vi "WaveFile_Create.vi"(0 "reference in":refnum<class "WaveFile.lvclass">, 5 "error in (no error)":errorcluster, 6 "Time Data":refnum<class "GSwFormDSP.lvclass">, 7 "Application Name":string, 9 "State Queue":string[](array[string])) -> (14 "reference out":refnum<class "WaveFile.lvclass">, 19 "error out":errorcluster)   [LabVIEW 2020, in "WaveFile.lvclass"]
doc: "Constructor."
uses:
  WaveFile.lvclass
  C:/Program Files/National Instruments/LabVIEW 2020/vi.lib/addons/_AddQ/G#Object/G#Object.lvclass
  C:/Users/fcharett/docsWork/coding/20SPWB/C/Users/fcharett/docsWork/coding/LabVIEW/API/Generic Utilities_class/Generic Utilities.lvclass
  API/GSwFormDSP_class/GSwFormDSP.lvclass
  <vilib>/addons/_AddQ/G#Object/G#Object.lvclass
  API/Generic Utilities_class/Generic Utilities.lvclass
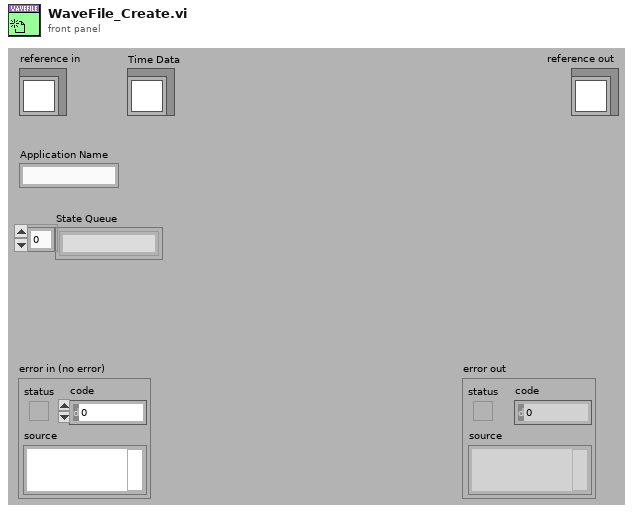
[diagram p1: front panel]
types:
  T1 = typedef "WaveFile.lvclass/ObjectAttributesRef.ctl" = refnum<data-value>
  T2 = typedef "WaveFile.lvclass/ObjectAttributes.ctl" = cluster{"Time Data":refnum<class "GSwFormDSP.lvclass">, "New Time Data Obj?":bool, "NIST File Header":T3}
  T3 = typedef "WaveFile.lvclass/NIST File Header.ctl" = cluster{"Version":string, "Header Nb Bytes":i32, "Nb Samples":i32, "Nb Bytes/sample":i32, "Nb Channels":i32, "byte order":enum16{"big-endian, network order", "native, host order", "little-endian"}, "Fs":dbl, "Valid Header?":bool}
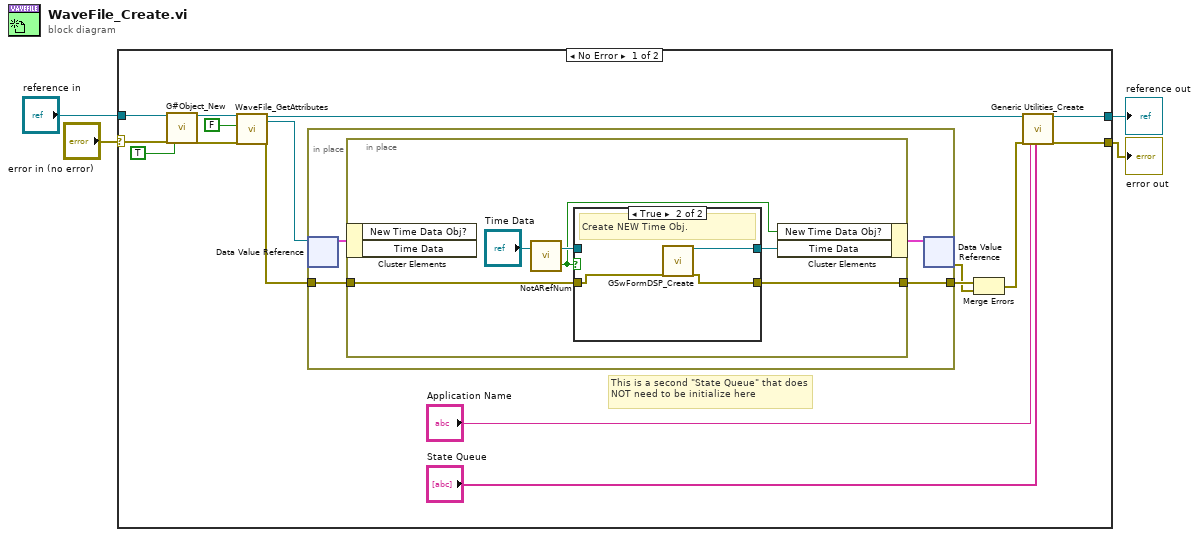
[diagram p0: block diagram]
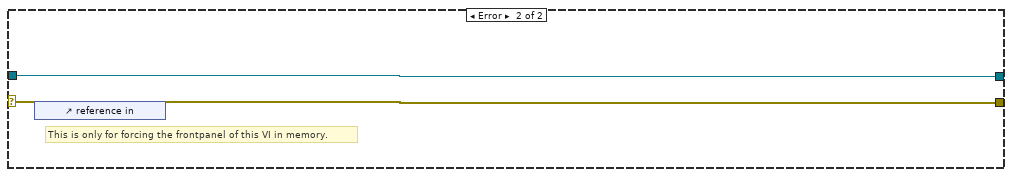
[diagram p3: hidden frame]
diagram:
  n1 = case shown="No Error" "error in (no error)" {
    selector: "error in (no error)" -> [w19 w37]
    tunnel: [w8 w37] -> w3
    tunnel: [w10 w36] -> w1
    tunnel: "reference in" -> [w20 w36]
    frame No Error {
      # "This is a second \"State Queue\" that does NOT need to be initialize here"
      n2 = call <vilib>:"G#Object_New.vi"("reference in"=w20, "error in (no error)"=w19, "user counter (T)?"=TRUE ("User Counter")) -> ("reference out"=w13:refnum<class "WaveFile.lvclass">, "error out"=w12:errorcluster)  [unwired: 14 in, 1 out]
      n3 = call "WaveFile_GetAttributes.vi"("reference in"=w13, "return data? (T)"=FALSE ("return data"), "error in (no error)"=w12) -> ("reference out"=w11:refnum<class "WaveFile.lvclass">, "attributes ref"=w15:T1, "error out"=w6:errorcluster)  [unwired: 13 in, 1 out]
      n4 = in-place {
        in-place-border: [w21] -> w17
        in-place-border: w6 -> [w22]
        n5 = in-place-dvr #1(w15) -> (w23:T2)  [unwired: 1 out]
        n6 = in-place {
          in-place-border: w22 -> [w27]
          in-place-border: [w26] -> w21
          n7 = in-place-cluster #2(w23) -> ()  [unwired: 2 out]
          n8 = call-dynamic "NotARefNum.vi"("reference in"="Time Data") -> ("not a refnum?"=w25:bool, "reference out"=w28:refnum<class "GSwFormDSP.lvclass">)  [unwired: 1 in]
          n9 = case shown="True" w25 {
            tunnel: [w32 w35] -> w29
            tunnel: w28 -> [w32 _]
            tunnel: w27 -> [w31 w34]
            tunnel: [w31 w33] -> w26
            frame False {
              # "Copy an existing reference."
            }
            frame True {
              # "Create NEW Time Obj."
              n10 = call "GSwFormDSP_Create.vi"("error in (no error)"=w34) -> ("reference out"=w35:refnum<class "GSwFormDSP.lvclass">, "error out"=w33:errorcluster)  [unwired: 17 in]
            }
          }
          n11 = in-place-cluster #2("New Time Data Obj?"=w25, "Time Data"=w29) -> (w24:T2)
        }
        n12 = in-place-dvr #1(w24) -> (w16:errorcluster)  [unwired: 1 out]
      }
      n13 = Merge Errors(w17, w16) -> (w9:errorcluster)
      n14 = call "Generic Utilities_Create.vi"("reference in"=w11, "error in (no error)"=w9, "Application Name"="Application Name", "State Queue"="State Queue") -> ("reference out"=w10:refnum<class "WaveFile.lvclass">, "error out"=w8:errorcluster)  [unwired: 14 in]
    }
    frame Error {
      # "This is only for forcing the frontpanel of this VI in memory."
      n15 = control-ref of="reference in"() -> ()  [unwired: 1 out]
    }
  }
  "error out" <- w3
  "reference out" <- w1
